vi "Convert From JSON Comp Format.vi"(8 "error in (no error)":errorcluster, 11 "input settings JSON":T1={"PDM clock rate"=51200.0, "decimation factor"=0.0, "bit clock direction"="", "logic level"=""} {"PDM clock rate" format="%#_6p"}) -> (0 "error out":errorcluster, 3 "input settings":T2={"PDM clock rate"=51200.0, "decimation factor"=1, "bit clock direction"=enum."In", "logic level"=enum."3.3 V"} {"decimation factor" items=["24"=24, "32"=32, "48"=48, "64"=64, "96"=96, "128"=128]; "PDM clock rate" format="%#_6p"})   [LabVIEW 2022 SP3, in "PDM input cfg file.lvlib"]
uses:
  PDM input cfg file.lvlib
  controls/PDM/PDM input settings.ctl
  <vilib>/PDM Acquisition Toolkit/shared/controls/decimation order.ctl
  controls/bit clock direction.ctl
  <vilib>/PDM Acquisition Toolkit/host/Classes/Session/Controls/Logic Levels.ctl
  controls/PDM/PDM input settings_json.ctl
  <vilib>/PDM Acquisition Toolkit/host/Classes/Session/DecoderSession.lvclass
  <vilib>/PDM Acquisition Toolkit/shared/PDM Shared.lvlib
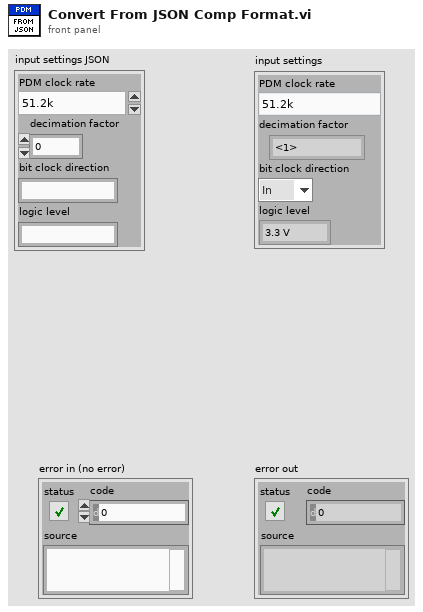
[diagram p1: front panel]
types:
  T1 = typedef "PDM input settings_json.ctl" = cluster{"PDM clock rate":dbl, "decimation factor":dbl, "bit clock direction":string, "logic level":string}
  T2 = typedef "PDM input settings.ctl" = cluster{"PDM clock rate":dbl, "decimation factor":T3, "bit clock direction":T4, "logic level":T5}
  T3 = typedef "PDM Shared.lvlib/decimation order.ctl" = u16
  T4 = typedef "bit clock direction.ctl" = enum32{"In", "Out"}
  T5 = typedef "PDM Acquisition Class Library.lvlib/DecoderSession.lvclass/Logic Levels.ctl" = enum16{"3.3 V", "1.8 V", "1.2 V"}
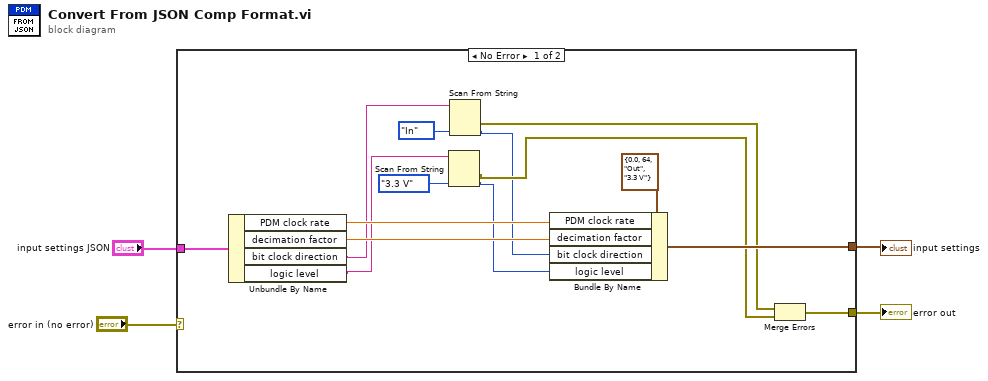
[diagram p0: block diagram]
diagram:
  n1 = case shown="No Error" "error in (no error)" {
    selector: "error in (no error)" -> [_ w19]
    tunnel: "input settings JSON" -> [w17 _]
    tunnel: [w16 _] -> w2
    tunnel: [w13 w19] -> w1
    frame No Error {
      n2 = Unbundle By Name(w17) -> ("PDM clock rate"=w12:dbl, "decimation factor"=w11:dbl, "bit clock direction"=w8:string, "logic level"=w7:string)
      n3 = Scan From String(input string=w7, default 1=Logic_Levels."3.3 V" ("logic level")) -> (error out=w14:errorcluster, output 1=w5:T5)  [unwired: 3 in, 2 out]
      n4 = Scan From String(input string=w8, default 1=bit_clock_direction."In" ("bit clock direction")) -> (error out=w15:errorcluster, output 1=w6:T4)  [unwired: 3 in, 2 out]
      n5 = Bundle By Name(cluster=T2 {"PDM clock rate"=0.0, "decimation factor"=64, "bit clock direction"=enum."Out", "logic level"=enum."3.3 V"} ("PDM input settings"), "PDM clock rate"=w12, "decimation factor"=w11, "bit clock direction"=w6, "logic level"=w5) -> (w16:T2)
      n6 = Merge Errors(w15, w14) -> (w13:errorcluster)
    }
    frame Error {
    }
  }
  "input settings" <- w2
  "error out" <- w1
